vi "HTML2DB.vi"(8 "error in (no error)":errorcluster) -> (0 "error out":errorcluster)   [LabVIEW 2012]
uses:
  <vilib>/addons/database/Connection.llb/DB Tools Open Connec (Path).vi
  <vilib>/addons/database/NI_Database_API.lvlib
panel:
  in  "input cluster 2":T1
  out "filenames":string[](array[string])
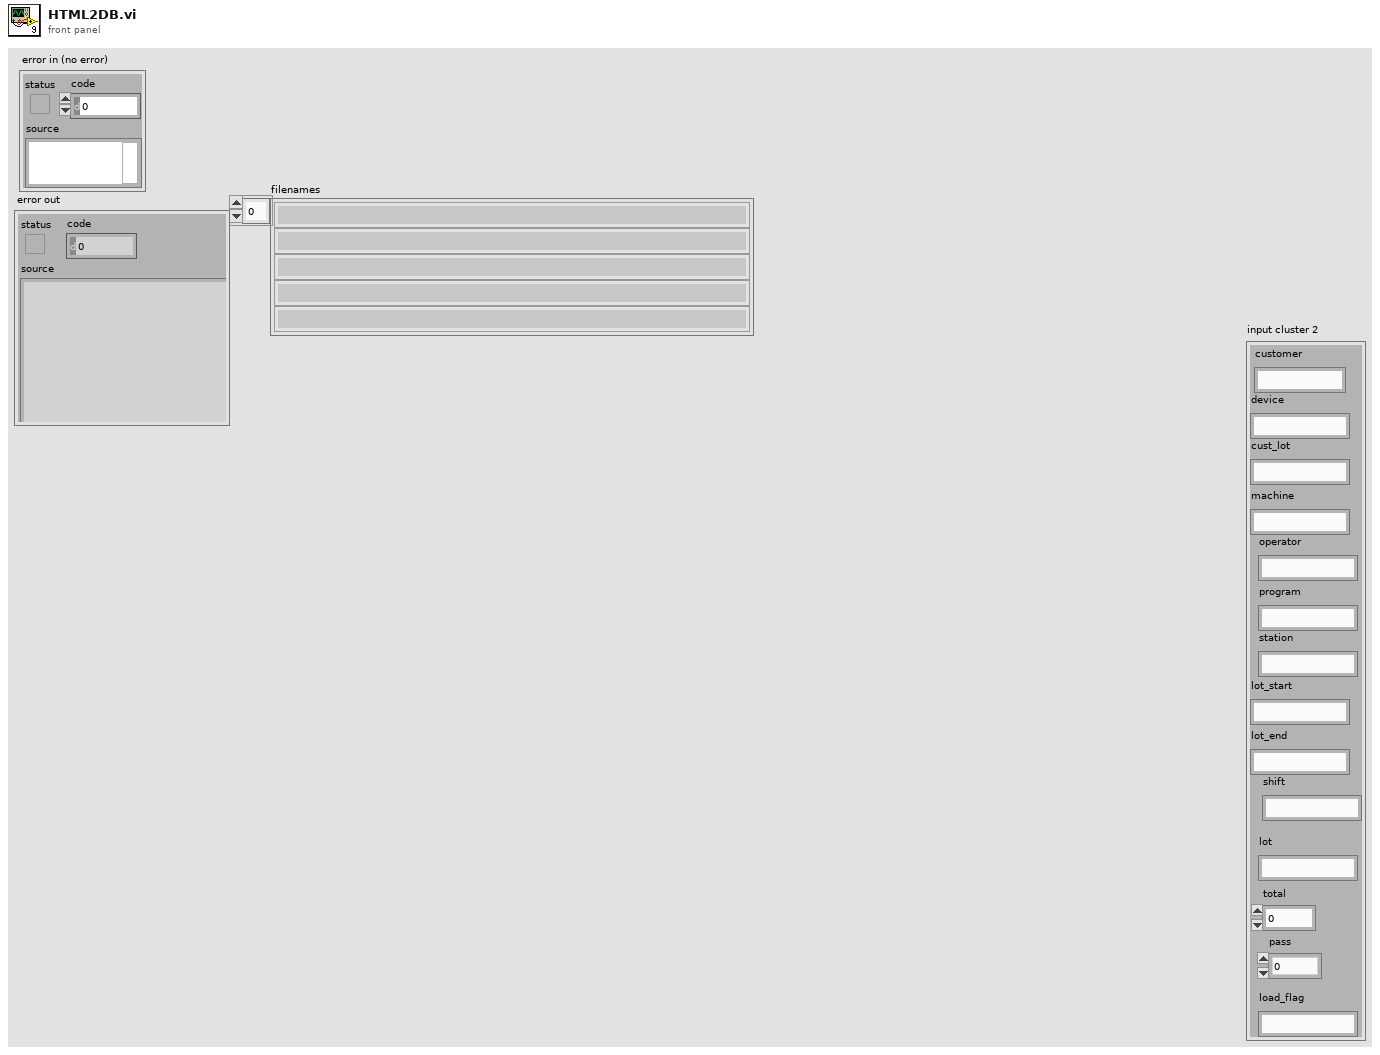
[diagram p1: front panel]
types:
  T1 = cluster{"customer":string, "device":string, "cust_lot":string, "machine":string, "operator":string, "program":string, "station":string, "lot_start":string, "lot_end":string, "shift":string, "lot":string, "total":dbl, "pass":dbl, "load_flag":string}
  T2 = typedef "NI_Database_API.lvlib/Conn ObjectReference.ctl" = refnum<k1>
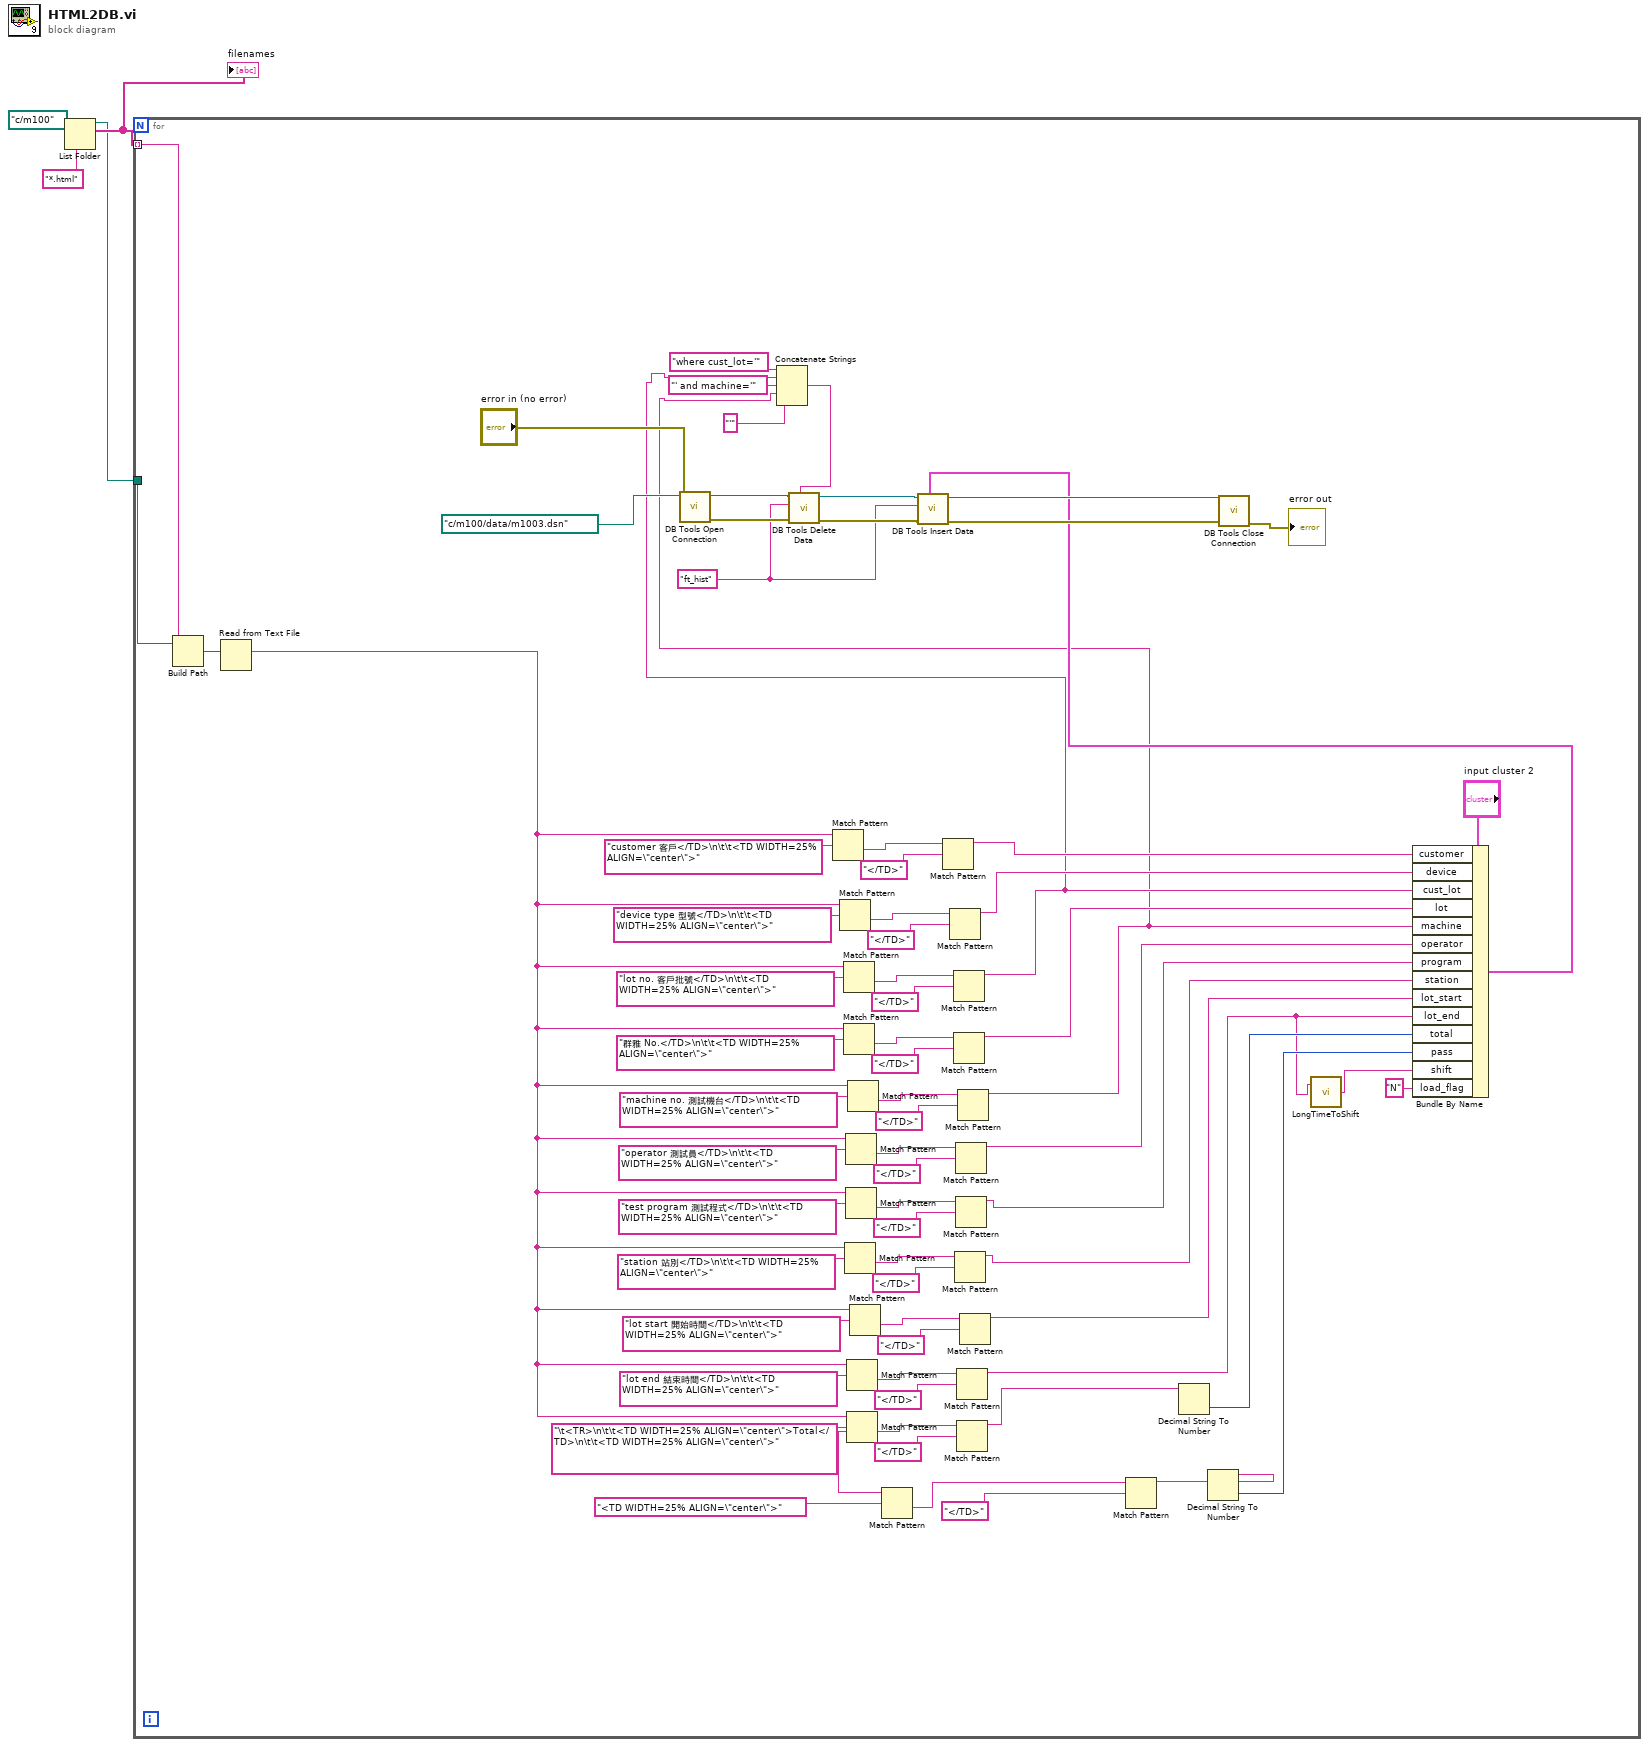
[diagram p0: block diagram]
diagram:
  n1 = List Folder(path=path "c:/m100", pattern="*.html") -> (path out=w1:path, filenames=w2:string[])  [unwired: 2 in, 2 out]
  "filenames" <- w2
  n2 = for {
    tunnel: w2 -> [w74] mode=indexing
    tunnel: w1 -> [w73]
    w12 = "ft_hist" ("table 2")
    n3 = Build Path(base path=w73, name or relative path=w74) -> (appended path=w75:path)
    n4 = Read from Text File(file (use dialog)=w75) -> (text=w40:string)  [unwired: 3 in, 3 out]
    n5 = call-poly <vilib>:"DB Tools Open Connection.vi"("error in (no error)"="error in (no error)", "connection information"=path "c:/m100/data/m1003.dsn") -> ("error out"=w14:errorcluster, "connection reference"=w16:T2)  [unwired: 6 in]
    n6 = Match Pattern(string=w40, regular expression="customer 客戶</TD>\n\t\t<TD WIDTH=25% ALIGN=\"center\">") -> (after substring=w71:string)  [unwired: 1 in, 3 out]
    n7 = Match Pattern(string=w40, regular expression="device type 型號</TD>\n\t\t<TD WIDTH=25% ALIGN=\"center\">") -> (after substring=w68:string)  [unwired: 1 in, 3 out]
    n8 = Match Pattern(string=w40, regular expression="lot no. 客戶批號</TD>\n\t\t<TD WIDTH=25% ALIGN=\"center\">") -> (after substring=w65:string)  [unwired: 1 in, 3 out]
    n9 = Match Pattern(string=w40, regular expression="群雅 No.</TD>\n\t\t<TD WIDTH=25% ALIGN=\"center\">") -> (after substring=w62:string)  [unwired: 1 in, 3 out]
    n10 = Match Pattern(string=w40, regular expression="station 站別</TD>\n\t\t<TD WIDTH=25% ALIGN=\"center\">") -> (after substring=w50:string)  [unwired: 1 in, 3 out]
    n11 = Match Pattern(string=w40, regular expression="operator 測試員</TD>\n\t\t<TD WIDTH=25% ALIGN=\"center\">") -> (after substring=w56:string)  [unwired: 1 in, 3 out]
    n12 = Match Pattern(string=w40, regular expression="test program 測試程式</TD>\n\t\t<TD WIDTH=25% ALIGN=\"center\">") -> (after substring=w53:string)  [unwired: 1 in, 3 out]
    n13 = Match Pattern(string=w40, regular expression="lot end 結束時間</TD>\n\t\t<TD WIDTH=25% ALIGN=\"center\">") -> (after substring=w44:string)  [unwired: 1 in, 3 out]
    n14 = Match Pattern(string=w40, regular expression="\t<TR>\n\t\t<TD WIDTH=25% ALIGN=\"center\">Total</TD>\n\t\t<TD WIDTH=25% ALIGN=\"center\">") -> (after substring=w39:string)  [unwired: 1 in, 3 out]
    n15 = Match Pattern(string=w40, regular expression="machine no. 測試機台</TD>\n\t\t<TD WIDTH=25% ALIGN=\"center\">") -> (after substring=w59:string)  [unwired: 1 in, 3 out]
    n16 = Match Pattern(string=w40, regular expression="lot start 開始時間</TD>\n\t\t<TD WIDTH=25% ALIGN=\"center\">") -> (after substring=w47:string)  [unwired: 1 in, 3 out]
    n17 = Match Pattern(string=w39, regular expression="<TD WIDTH=25% ALIGN=\"center\">") -> (after substring=w36:string)  [unwired: 1 in, 3 out]
    n18 = Match Pattern(string=w71, regular expression="</TD>") -> (before substring=w31:string)  [unwired: 1 in, 3 out]
    n19 = Match Pattern(string=w68, regular expression="</TD>") -> (before substring=w30:string)  [unwired: 1 in, 3 out]
    n20 = Match Pattern(string=w65, regular expression="</TD>") -> (before substring=w10:string)  [unwired: 1 in, 3 out]
    n21 = Match Pattern(string=w62, regular expression="</TD>") -> (before substring=w29:string)  [unwired: 1 in, 3 out]
    n22 = Match Pattern(string=w50, regular expression="</TD>") -> (before substring=w26:string)  [unwired: 1 in, 3 out]
    n23 = Match Pattern(string=w56, regular expression="</TD>") -> (before substring=w28:string)  [unwired: 1 in, 3 out]
    n24 = Match Pattern(string=w53, regular expression="</TD>") -> (before substring=w27:string)  [unwired: 1 in, 3 out]
    n25 = Match Pattern(string=w44, regular expression="</TD>") -> (before substring=w22:string)  [unwired: 1 in, 3 out]
    n26 = Match Pattern(string=w39, regular expression="</TD>") -> (before substring=w35:string)  [unwired: 1 in, 3 out]
    n27 = Match Pattern(string=w59, regular expression="</TD>") -> (before substring=w8:string)  [unwired: 1 in, 3 out]
    n28 = Concatenate Strings("where cust_lot='" ("string"), w10, "' and machine='" ("string"), w8, "'" ("string")) -> (w6:string)
    n29 = call <vilib>:"DB Tools Delete Data.vi"("condition"=w6, "error in (no error)"=w14, "table"=w12, "connection reference"=w16) -> ("error out"=w13:errorcluster, "connection reference out"=w15:T2)  [unwired: 6 in]
    n30 = Match Pattern(string=w47, regular expression="</TD>") -> (before substring=w25:string)  [unwired: 1 in, 3 out]
    n31 = Match Pattern(string=w36, regular expression="</TD>") -> (before substring=w34:string)  [unwired: 1 in, 3 out]
    n32 = Decimal String To Number(string=w35) -> (number=w24:i32)  [unwired: 2 in, 1 out]
    n33 = Decimal String To Number(string=w34) -> (number=w23:i32)  [unwired: 2 in, 1 out]
    n34 = call "LongTimeToShift.vi"("input string"=w22) -> ("s? t:f"=w21:string)  [unwired: 1 in]
    n35 = Bundle By Name(cluster="input cluster 2", "customer"=w31, "device"=w30, "cust_lot"=w10, "lot"=w29, "machine"=w8, "operator"=w28, "program"=w27, "station"=w26, "lot_start"=w25, "lot_end"=w22, "total"=w24, "pass"=w23, "shift"=w21, "load_flag"="N") -> (w18:T1)
    n36 = call <vilib>:"DB Tools Insert Data.vi"("data"=w18, "error in (no error)"=w13, "table"=w12, "connection reference"=w15) -> ("error out"=w19:errorcluster, "connection reference out"=w20:T2)  [unwired: 6 in]
    n37 = call <vilib>:"DB Tools Close Connection.vi"("error in (no error)"=w19, "connection reference"=w20) -> ("error out"=→"error out":errorcluster)  [unwired: 5 in]
  }
